vi "GetIntervalTime.vi"(8 "error in":errorcluster, 11 "VISA resource name":refnum<visa-resource-name>) -> (0 "error out":errorcluster, 2 "Interval Time":string, 3 "VISA resource name out":refnum<visa-resource-name>)   [LabVIEW 2023, in "Thermotron 8800.lvlib"]
doc: "ITIM\nCommand name: Send interval time\nCommand type: Program status\nDescription: Queries the 8800 for the programmed time for the current interval.\nSyntax: ITIM?\nData type: String\nQuery example: ITIM?\n8800 response: 0:10:30 (The current interval is 10 minutes, 30 seconds long.)"
uses:
  Thermotron 8800.lvlib
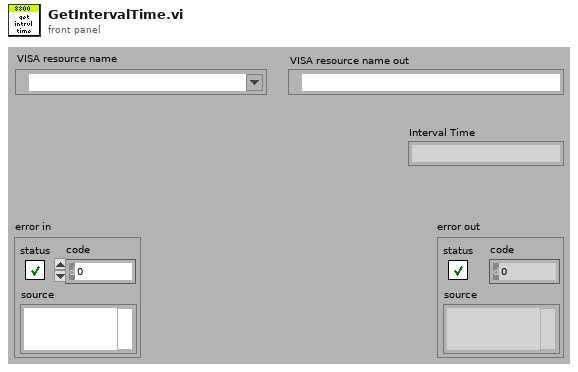
[diagram p1: front panel]
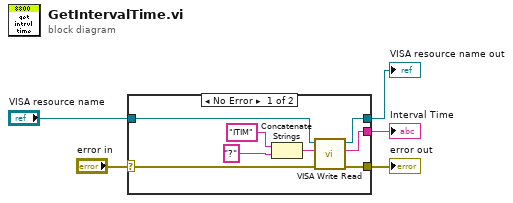
[diagram p0: block diagram]
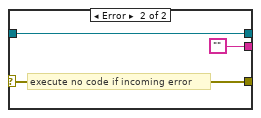
[diagram p2: hidden frame]
diagram:
  n1 = case shown="No Error" "error in" {
    selector: "error in" -> [w12 w16]
    tunnel: [w10 w16] -> w2
    tunnel: [w11 w15] -> w3
    tunnel: "VISA resource name" -> [w8 w15]
    tunnel: [w6 ""] -> w1
    frame No Error {
      n2 = Concatenate Strings("ITIM" ("8800 Command"), "?" ("8800 Command")) -> (w13:string)
      n3 = call "VISA Write Read.vi"("error in (no error)"=w12, "8800 Command"=w13, "VISA Refnum in"=w8) -> ("error out"=w10:errorcluster, "read buffer"=w6:string, "VISA Refnum out"=w11:refnum<visa-resource-name>)  [unwired: 6 in]
    }
    frame Error {
      # "execute no code if incoming error"
    }
  }
  "VISA resource name out" <- w3
  "error out" <- w2
  "Interval Time" <- w1
